vi "Process Clock.vi"(11 "IO in":refnum<class "IO.lvclass">) -> (3 "IO out":refnum<class "IO.lvclass">)   [LabVIEW 2021, in "IO.lvclass"]
uses:
  IO.lvclass
  IO.lvclass/IO.ctl
  Memory Map/Memory Map.lvclass
  Memory/Memory.lvclass
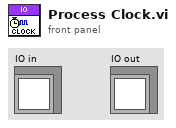
[diagram p1: front panel]
types:
  T1 = typedef "Memory Map.lvclass/Active Device.ctl" = enum16{"Error", "None", "RAM", "EEPROM", "VIA"}
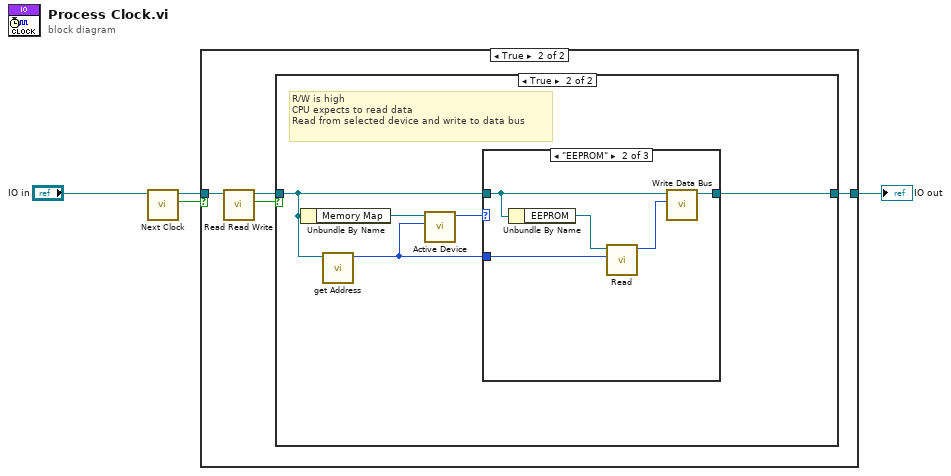
[diagram p0: block diagram]
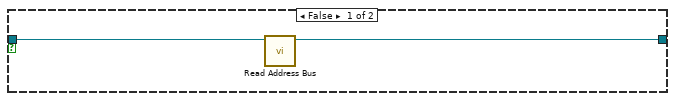
[diagram p2: hidden frame]
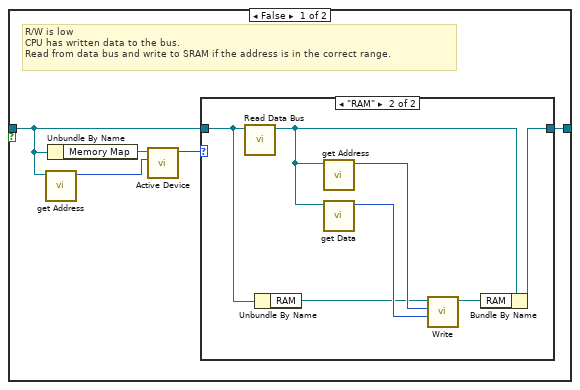
[diagram p3: hidden frame]
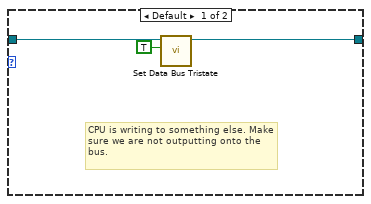
[diagram p4: hidden frame]
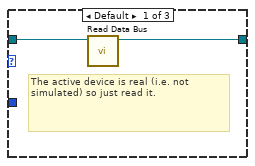
[diagram p5: hidden frame]
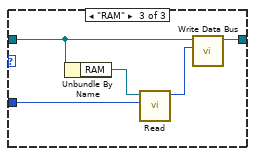
[diagram p6: hidden frame]
diagram:
  n1 = call "Next Clock.vi"("Clock Generator in"="IO in") -> ("Current State"=w2:bool, "Clock Generator out"=w3:refnum<class "IO.lvclass">)  [unwired: 8 in, 1 out]
  n2 = case shown="True" w2 {
    tunnel: w3 -> [w6 w8]
    tunnel: [w5 w10] -> w4
    frame False {
      n3 = call "Read Address Bus.vi"("IO in"=w6) -> ("IO out"=w5:refnum<class "IO.lvclass">)  [unwired: 9 in, 1 out]
    }
    frame True {
      n4 = call "Read Read Write.vi"("IO in"=w8) -> ("R/W"=w7:bool, "IO out"=w9:refnum<class "IO.lvclass">)  [unwired: 8 in, 1 out]
      n5 = case shown="True" w7 {
        tunnel: w9 -> [w13 w27]
        tunnel: [w15 w30] -> w10
        frame False {
          # "R/W is low\nCPU has written data to the bus. \nRead from data bus and write to SRAM if the address is in the correct range."
          n6 = call "get Address.vi"("IO in"=w13) -> ("Address"=w12:u16)  [unwired: 10 in]
          n7 = Unbundle By Name(w13) -> ("Memory Map"=w14:refnum<class "Memory Map.lvclass">)
          n8 = call "Active Device.vi"("Address"=w12, "Memory Map in"=w14) -> ("Active Device"=w11:T1)  [unwired: 9 in]
          n9 = case shown="\"RAM\"" w11 {
            tunnel: [w18 w22] -> w15
            tunnel: w13 -> [w17 w19]
            frame Default {
              # "CPU is writing to something else. Make sure we are not outputting onto the bus."
              n10 = call "Set Data Bus Tristate.vi"("Tristate"=TRUE, "IO in"=w17) -> ("IO out"=w18:refnum<class "IO.lvclass">)  [unwired: 8 in, 1 out]
            }
            frame "RAM" {
              n11 = call "Read Data Bus.vi"("IO in"=w19) -> ("IO out"=w23:refnum<class "IO.lvclass">)  [unwired: 9 in, 1 out]
              n12 = Unbundle By Name(w19) -> ("RAM"=w20:refnum<class "Memory.lvclass">)
              n13 = call "get Address.vi"("IO in"=w23) -> ("Address"=w25:u16)  [unwired: 10 in]
              n14 = call "get Data.vi"("IO in"=w23) -> ("Data"=w24:u8)  [unwired: 10 in]
              n15 = call "Write.vi"("Data"=w24, "Address"=w25, "Memory in"=w20) -> ("Memory out"=w21:refnum<class "Memory.lvclass">)  [unwired: 8 in]
              n16 = Bundle By Name(cluster=w23, "RAM"=w21) -> (w22:refnum<class "IO.lvclass">)
            }
          }
        }
        frame True {
          # "R/W is high\nCPU expects to read data\nRead from selected device and write to data bus"
          n17 = Unbundle By Name(w27) -> ("Memory Map"=w26:refnum<class "Memory Map.lvclass">)
          n18 = call "get Address.vi"("IO in"=w27) -> ("Address"=w28:u16)  [unwired: 10 in]
          n19 = call "Active Device.vi"("Address"=w28, "Memory Map in"=w26) -> ("Active Device"=w29:T1)  [unwired: 9 in]
          n20 = case shown="\"EEPROM\"" w29 {
            tunnel: [w31 w37 w42] -> w30
            tunnel: w27 -> [w32 w34 w39]
            tunnel: w28 -> [_ w35 w40]
            frame Default {
              # "The active device is real (i.e. not simulated) so just read it."
              n21 = call "Read Data Bus.vi"("IO in"=w32) -> ("IO out"=w31:refnum<class "IO.lvclass">)  [unwired: 9 in, 1 out]
            }
            frame "EEPROM" {
              n22 = Unbundle By Name(w34) -> ("EEPROM"=w33:refnum<class "Memory.lvclass">)
              n23 = call "Read.vi"("Address"=w35, "Memory in"=w33) -> ("Data"=w36:u8)  [unwired: 9 in]
              n24 = call "Write Data Bus.vi"("Data"=w36, "IO in"=w34) -> ("IO out"=w37:refnum<class "IO.lvclass">)  [unwired: 8 in, 1 out]
            }
            frame "RAM" {
              n25 = Unbundle By Name(w39) -> ("RAM"=w38:refnum<class "Memory.lvclass">)
              n26 = call "Read.vi"("Address"=w40, "Memory in"=w38) -> ("Data"=w41:u8)  [unwired: 9 in]
              n27 = call "Write Data Bus.vi"("Data"=w41, "IO in"=w39) -> ("IO out"=w42:refnum<class "IO.lvclass">)  [unwired: 8 in, 1 out]
            }
          }
        }
      }
    }
  }
  "IO out" <- w4
